vi "NGTS_DAQmx Analog Create Custom Scales.vi"(8 "error in":errorcluster, 9 "Save As Global Channel":bool, 10 "Author":string="Mike Ashe", 11 "Channels Properties Table":string[][](array[string])) -> (0 "error out":errorcluster, 2 "Custom Scales":tag[](array[tag]), 3 "Custom Scale Names":string[](array[string]))   [LabVIEW 2018]
doc: "Parses rows in the Channel Properties Table and creates custom scales for the Voltage and Amperage types. Thermocouples (denoted by using \"deg\" in the units) are not scaled here.\n\n2007-11 Mike Ashe\nmichael.ashe@imaginatics.net\nCell: 860-961-0876"
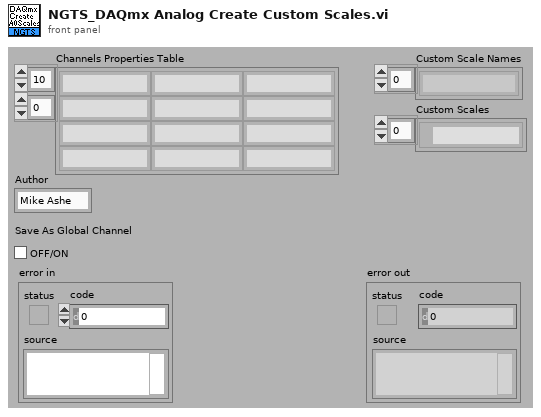
[diagram p1: front panel]
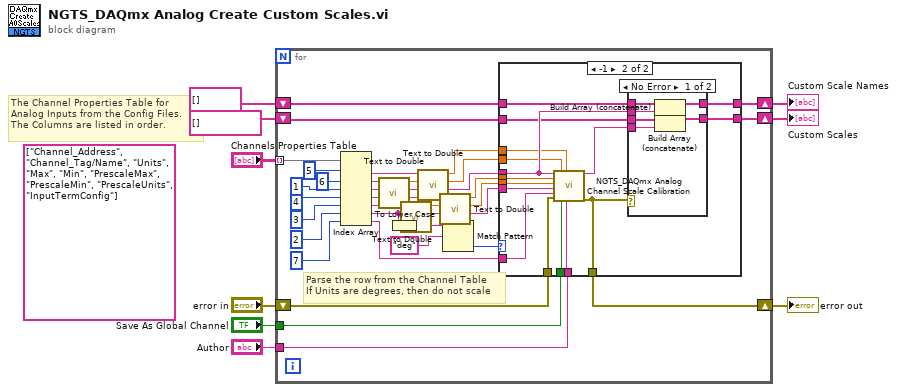
[diagram p0: block diagram]
diagram:
  (unwired) string[] ["Channel_Address", "Channel_Tag/Name", "Units", "Max", "Min", "PrescaleMax", "PrescaleMin", "PrescaleUnits", "InputTermConfig"]
  # "The Channel Properties Table for\nAnalog Inputs from the Config Files.\nThe Columns are listed in order."
  n1 = for {
    tunnel: "Channels Properties Table" -> [w39] mode=indexing
    tunnel: "Author" -> [w36]
    tunnel: "Save As Global Channel" -> [w35]
    shift-right: [w31] -> w3
    shift-left: string[] [] -> [w29]
    shift-right: [w30] -> w4
    shift-left: tag[] [] -> [w28]
    shift-right: [w26] -> w1
    shift-left: "error in" -> [w27]
    # "Parse the row from the Channel Table\nIf Units are degrees, then do not scale"
    n2 = Index Array(array=w39, index #1=5 ("index"), index #2=6 ("index"), index #3=1 ("index"), index #4=4 ("index"), index #5=3 ("index"), index #6=2 ("index"), index #7=7 ("index")) -> (element #1=w13:string, element #2=w14:string, element #3=w17:string, element #4=w18:string, element #5=w20:string, element #6=w23:string, element #7=w24:string)
    n3 = call "Text to Double.vi"("string"=w14) -> ("number"=w11:dbl)  [unwired: 10 in]
    n4 = To Lower Case(string=w23) -> (all lower case string=w34:string)
    n5 = call "Text to Double.vi"("string"=w20) -> ("number"=w37:dbl)  [unwired: 10 in]
    n6 = call "Text to Double.vi"("string"=w13) -> ("number"=w10:dbl)  [unwired: 10 in]
    n7 = call "Text to Double.vi"("string"=w18) -> ("number"=w38:dbl)  [unwired: 10 in]
    n8 = Match Pattern(string=w34, regular expression="deg") -> (offset past match=w32:i32)  [unwired: 1 in, 3 out]
    n9 = case shown="-1" w32 {
      tunnel: w17 -> [_ w51]
      tunnel: w38 -> [_ w58]
      tunnel: w37 -> [_ w57]
      tunnel: w36 -> [_ w46]
      tunnel: w35 -> [_ w56]
      tunnel: w23 -> [_ w55]
      tunnel: [w42 w54] -> w31
      tunnel: [w41 w53] -> w30
      tunnel: w29 -> [w42 w52]
      tunnel: w28 -> [w41 w49]
      tunnel: w27 -> [w40 w48]
      tunnel: [w40 w47] -> w26
      tunnel: w24 -> [_ w45]
      tunnel: w11 -> [_ w44]
      tunnel: w10 -> [_ w43]
      frame 0, Default {
      }
      frame -1 {
        n10 = call "NGTS_DAQmx Analog Channel Scale Calibration.vi"("Scale Identifier"=w51, "scaled min"=w58, "scaled max"=w57, "scaled units"=w55, "prescaled units"=w45, "error in"=w48, "prescaled min"=w44, "Save As Global Channel"=w56, "prescaled max"=w43, "Author"=w46) -> ("Custom Scale Out"=w50:tag, "error out"=w47:errorcluster)  [unwired: 8 in]
        n11 = case shown="No Error" w47 {
          tunnel: [w64 w66] -> w54
          tunnel: [w63 w65] -> w53
          tunnel: w52 -> [w62 w66]
          tunnel: w51 -> [w61 _]
          tunnel: w50 -> [w60 _]
          tunnel: w49 -> [w59 w65]
          frame No Error {
            n12 = Build Array (concatenate)(w62, w61) -> (w64:string[])
            n13 = Build Array (concatenate)(w59, w60) -> (w63:tag[])
          }
          frame Error {
          }
        }
      }
    }
  }
  "Custom Scales" <- w4
  "Custom Scale Names" <- w3
  "error out" <- w1
